vi "RIO_I2C_PmodGYROClose.vi"(8 "error in (no error)":errorcluster, 10 "refnum name":string="My I2C RefNum") -> (0 "error out":errorcluster)   [LabVIEW 2018]
doc: "Close the specified I2C channel."
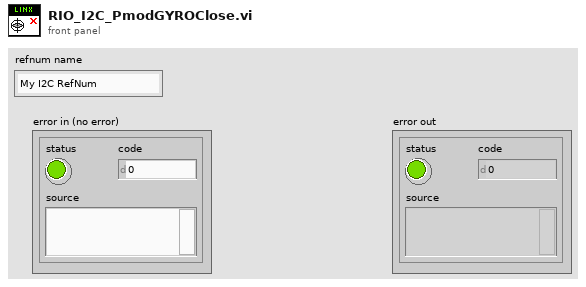
[diagram p1: front panel]
types:
  T1 = typedef "WPI_I2CDevRef.ctl" = cluster{"DevStatus":errorcluster, "Device Address":u8, "Handle":i32, "I2C Bus":T2}
  T2 = typedef "i2c_bus.ctl" = enum16{"I2C On-Board", "I2C MXP", "Invalid"}
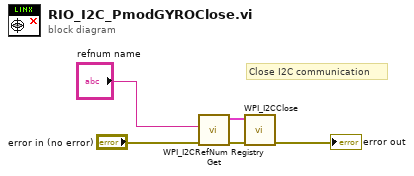
[diagram p0: block diagram]
diagram:
  # "Close I2C communication"
  n1 = call <vilib>:"WPI_I2CRefNum Registry Get.vi"("error in (no error)"="error in (no error)", "refnum name"="refnum name") -> ("error out"=w4:errorcluster, "I2CDevRef"=w5:T1)  [unwired: 8 in]
  n2 = call <vilib>:"WPI_I2CClose.vi"("error in (no error)"=w4, "I2CDevRef"=w5) -> ("error out"=→"error out":errorcluster)  [unwired: 9 in]
